vi "Set_speed_and_move_Y.vi"() -> ()   [LabVIEW 2013]
panel:
  out "Received String2":string="R\r\n"
  out "String Received 2":string="OK\r\n"
  out "Command String 2":string="A:2+P100"
  out "OK move 1":bool=TRUE
  in  "Pulse Number 1":u32=100 min=1 max=500000
  in  "Axis Number 1":u8=2
  out "OK speed 1":bool=TRUE
  in  "Port Number":i8=7 min=0
  out "String Received":string="OK\r\n"
  out "Command String":string="D:2S1000F10000R100"
  in  "Acceleration Time":u16=100 max=1000
  in  "High Speed":u32=10000 min=1 max=500000
  in  "Low Speed":u32=1000 min=1 max=500000
  # "For tensile test (30 mm sample length):\nSet local origin as X (axis 1) 27000, Y (axis 2) 5000"
  # "Set speed"
  # "Move to the absolute position"
  # "Abs. position X\nin um"
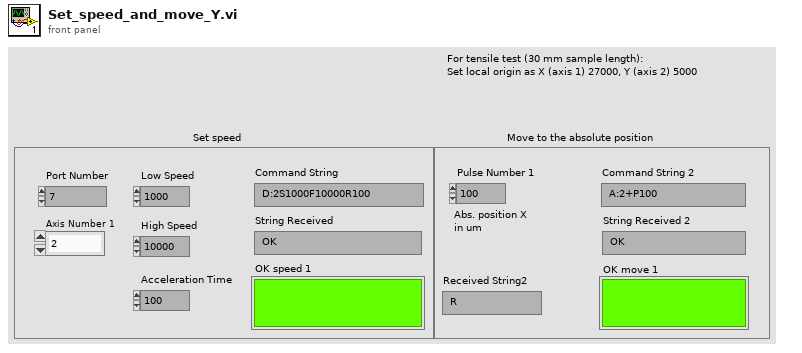
[diagram p1: front panel]
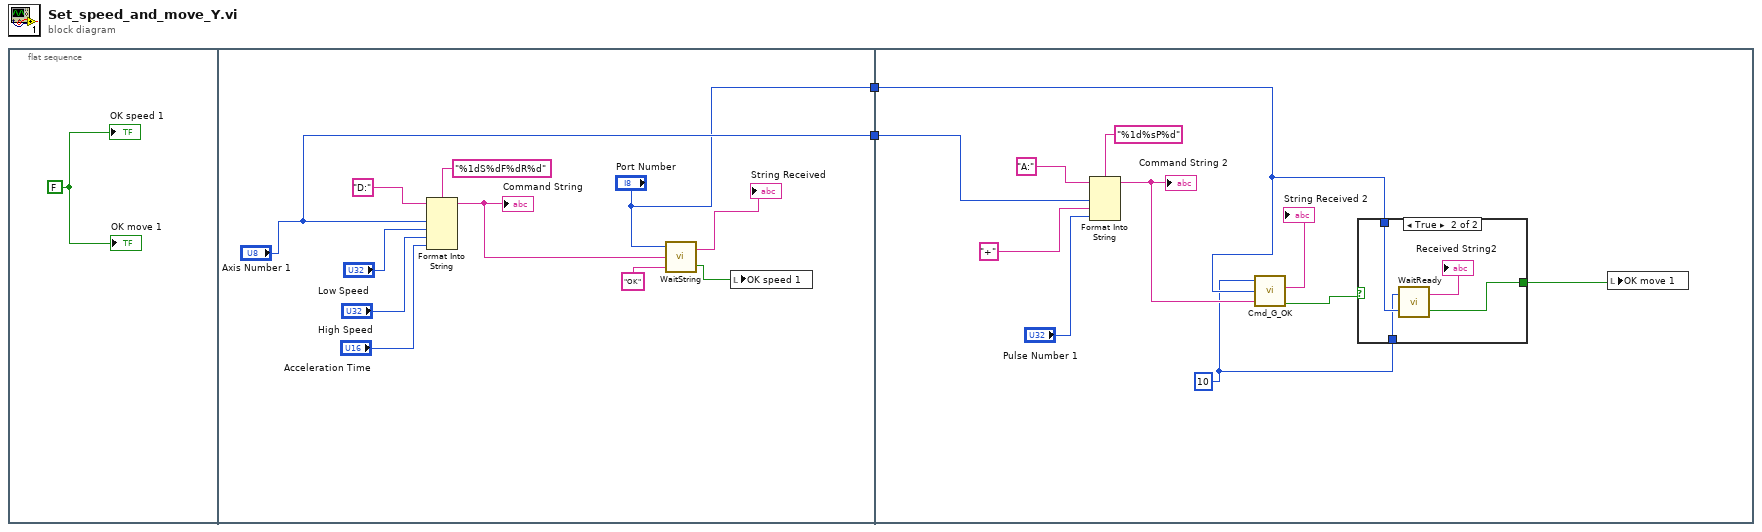
[diagram p0: block diagram]
diagram:
  n1 = flat-sequence {
    tunnel: ["Axis Number 1"] -> w2
    tunnel: ["Port Number"] -> w1
    tunnel: w2 -> [w18]
    tunnel: w1 -> [w17]
    frame #0 {
      w3 = FALSE
      "OK speed 1" <- w3
      "OK move 1" <- w3
    }
    frame #1 {
      n2 = Format Into String(format string="%1dS%dF%dR%d", initial string="D:", "Axis Number 1", "Low Speed", "High Speed", "Acceleration Time") -> (resulting string=w8:string)  [unwired: 1 in, 1 out]
      "Command String" <- w8
      n3 = call "WaitString.vi"("String to Receive"="OK", "String to Send"=w8, "PortNumber"="Port Number") -> ("OK Done"=w4:bool, "String Received"=→"String Received":string)
      n4 = local write "OK speed 1"(w4) -> ()
    }
    frame #2 {
      w15 = 10
      n5 = Format Into String(format string="%1d%sP%d", initial string="A:", w18, "+", "Pulse Number 1") -> (resulting string=w22:string)  [unwired: 1 in, 1 out]
      "Command String 2" <- w22
      n6 = call "Cmd_G_OK.vi"("Residence time"=w15, "PortNumber"=w17, "Command String"=w22) -> ("Received String2"=→"String Received 2":string, "OK Done"=w24:bool)  [unwired: 2 out]
      n7 = case shown="True" w24 {
        selector: w24 -> [w26 _]
        tunnel: w17 -> [_ w30]
        tunnel: [w26 w28] -> w16
        tunnel: w15 -> [_ w27]
        frame False {
        }
        frame True {
          n8 = call "WaitReady.vi"("PortNumber"=w30, "Residence time in ms"=w27) -> ("OK Done"=w28:bool, "String Received"=→"Received String2":string)
        }
      }
      n9 = local write "OK move 1"(w16) -> ()
    }
  }
